vi "channels_to_stream.get.vi"(8 "error in (no error)":errorcluster, 11 "Nominal IO Client in":T1 format="%.0x") -> (0 "error out":errorcluster, 2 "Channels to Stream":string[](array[string]), 3 "Nominal IO Client out":T1 format="%.0x", 4 "Replaced":bool)   [LabVIEW 2024, in "Nominal IO VeriStand Client Scripting.lvlib"]
uses:
  <vilib>/NI VeriStand/Custom Device API/Custom Device Item Ref.ctl
  Nominal IO VeriStand Client Scripting.lvlib
  <vilib>/NI VeriStand/Custom Device API/Custom Device API.lvlib
  <vilib>/NI VeriStand/Custom Device API/Get Item Property (String Array).vi
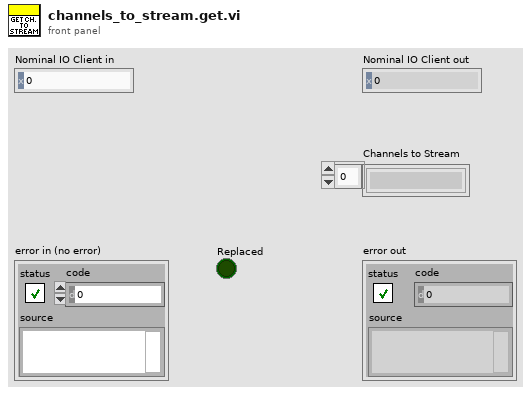
[diagram p1: front panel]
types:
  T1 = typedef "Custom Device API.lvlib/Custom Device Item Ref.ctl" = u64
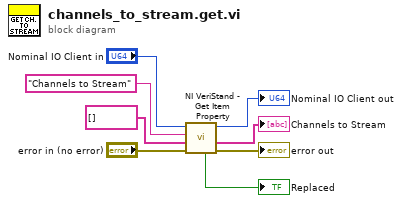
[diagram p0: block diagram]
diagram:
  n1 = call-poly <vilib>:"NI VeriStand - Get Item Property.vi"("error in (no error)"="error in (no error)", "Default Value"=string[] [] ("Property Name"), "Property Name"="Channels to Stream", "Item Ref in"="Nominal IO Client in") -> ("error out"=→"error out":errorcluster, "Value"=→"Channels to Stream":string[], "Item Ref out"=→"Nominal IO Client out":T1, "Found?"=→"Replaced":bool)  [unwired: 4 in]
